vi "toml_example_load.vi"(8 "error in (no error)":errorcluster) -> (0 "error out":errorcluster)   [LabVIEW 2017]
panel:
  out "tables":variant
  in  "toml":string="################################################################################\n## Comment\n\n# Speak your mind with the hash symbol. They go from the symbol to the end of\n# the line.\n\n\n################################################################################\n## Table\n\n# Tables (also known as hash tables or dictionaries) are collections of\n# key/value pairs. They appear in square brackets on a line by themselves.\n\n[table]\n\nkey = \"value\" # Yeah, you can do this.\n\n# Nested tables are denoted by table names with dots in them. Name your tables\n# whatever crap you please, just don't use #, ., [ or ].\n\n[table.subtable]\n\nkey = \"another value\"\n\n# You don't need to specify all the super-tables if you don't want to. TOML\n# knows how to do it for you.\n\n# [x] you\n# [x.y] don't\n# [x.y.z] need these\n[x.y.z.w] # for this to work\n\n\n################################################################################\n## Inline Table\n\n# Inline tables provide a more compact syntax for expressing tables. They are\n# especially useful for grouped data that can otherwise quickly become verbose.\n# Inline tables are enclosed in curly braces `{` and `}`. No newlines are\n# allowed between the curly braces unless they are valid within a value.\n\n[table.inline]\n\nname = { first = \"Tom\", last = \"Preston-Werner\" }\npoint = { x = 1, y = 2 }\n\n\n################################################################################\n## String\n\n# There are four ways to express strings: basic, multi-line basic, literal, and\n# multi-line literal. All strings must contain only valid UTF-8 characters.\n\n[string.basic]\n\nbasic = \"I'm a string. \\\"You can quote me\\\". Name\\tJos\\u00E9\\nLocation\\tSF.\"\n\n[string.multiline]\n\n# The following strings are byte-for-byte equivalent:\nkey1 = \"One\\nTwo\"\nkey2 = \"\"\"One\\nTwo\"\"\"\nkey3 = \"\"\"\nOne\nTwo\"\"\"\n\n[string.multiline.continued]\n\n# The following strings are byte-for-byte equivalent:\nkey1 = \"The quick brown fox jumps over the lazy dog.\"\n\nkey2 = \"\"\"\nThe quick brown \\\n\n\n  fox jumps over \\\n    the lazy dog.\"\"\"\n\nkey3 = \"\"\"\\\n       The quick brown \\\n       fox jumps over \\\n       the lazy dog.\\\n       \"\"\"\n\n[string.literal]\n\n# What you see is what you get.\nwinpath  = 'C:\\Users\\nodejs\\templates'\nwinpath2 = '\\\\ServerX\\admin$\\system32\\'\nquoted   = 'Tom \"Dubs\" Preston-Werner'\nregex    = '<\\i\\c*\\s*>'\n\n\n[string.literal.multiline]\n\nregex2 = '''I [dw]on't need \\d{2} apples'''\nlines  = '''\nThe first newline is\ntrimmed in raw strings.\n   All other whitespace\n   is preserved.\n'''\n\n\n################################################################################\n## Integer\n\n# Integers are whole numbers. Positive numbers may be prefixed with a plus sign.\n# Negative numbers are prefixed with a minus sign.\n\n[integer]\n\nkey1 = +99\nkey2 = 42\nkey3 = 0\nkey4 = -17\n\n[integer.underscores]\n\n# For large numbers, you may use underscores to enhance readability. Each\n# underscore must be surrounded by at least one digit.\nkey1 = 1_000\nkey2 = 5_349_221\nkey3 = 1_2_3_4_5     # valid but inadvisable\n\n\n################################################################################\n## Float\n\n# A float consists of an integer part (which may be prefixed with a plus or\n# minus sign) followed by a fractional part and/or an exponent part.\n\n[float.fractional]\n\nkey1 = +1.0\nkey2 = 3.1415\nkey3 = -0.01\n\n[float.exponent]\n\nkey1 = 5e+22\nkey2 = 1e6\nkey3 = -2E-2\n\n[float.both]\n\nkey = 6.626e-34\n\n[float.underscores]\n\nkey1 = 9_224_617.445_991_228_313\nkey2 = 1e1_000\n\n\n################################################################################\n## Boolean\n\n# Booleans are just the tokens you're used to. Always lowercase.\n\n[boolean]\n\nTrue = true\nFalse = false\n\n\n################################################################################\n## Datetime\n\n# Datetimes are RFC 3339 dates.\n\n[datetime]\n\nkey1 = 1979-05-27T07:32:00Z\nkey2 = 1979-05-27T00:32:00-07:00\nkey3 = 1979-05-27T00:32:00.999999-07:00\n\n\n################################################################################\n## Array\n\n# Arrays are square brackets with other primitives inside. Whitespace is\n# ignored. Elements are separated by commas. Data types may not be mixed.\n\n[array]\n\nkey1 = [ 1, 2, 3 ]\nkey2 = [ \"red\", \"yellow\", \"green\" ]\nkey3 = [ [ 1, 2 ], [3, 4, 5] ]\nkey4 = [ [ 1, 2 ], [\"a\", \"b\", \"c\"] ] # this is ok\n\n# Arrays can also be multiline. So in addition to ignoring whitespace, arrays\n# also ignore newlines between the brackets.  Terminating commas are ok before\n# the closing bracket.\n\nkey5 = [\n  1, 2, 3\n]\nkey6 = [\n  1,\n  2, # this is ok\n]\n\n\n################################################################################\n## Array of Tables\n\n# These can be expressed by using a table name in double brackets. Each table\n# with the same double bracketed name will be an element in the array. The\n# tables are inserted in the order encountered.\n\n[[products]]\n\nname = \"Hammer\"\nsku = 738594937\n\n[[products]]\n\n[[products]]\n\nname = \"Nail\"\nsku = 284758393\ncolor = \"gray\"\n\n\n# You can create nested arrays of tables as well.\n\n[[fruit]]\n  name = \"apple\"\n\n  [fruit.physical]\n    color = \"red\"\n    shape = \"round\"\n\n  [[fruit.variety]]\n    name = \"red delicious\"\n\n  [[fruit.variety]]\n    name = \"granny smith\"\n\n[[fruit]]\n  name = \"banana\"\n\n  [[fruit.variety]]\n    name = \"plantain\""
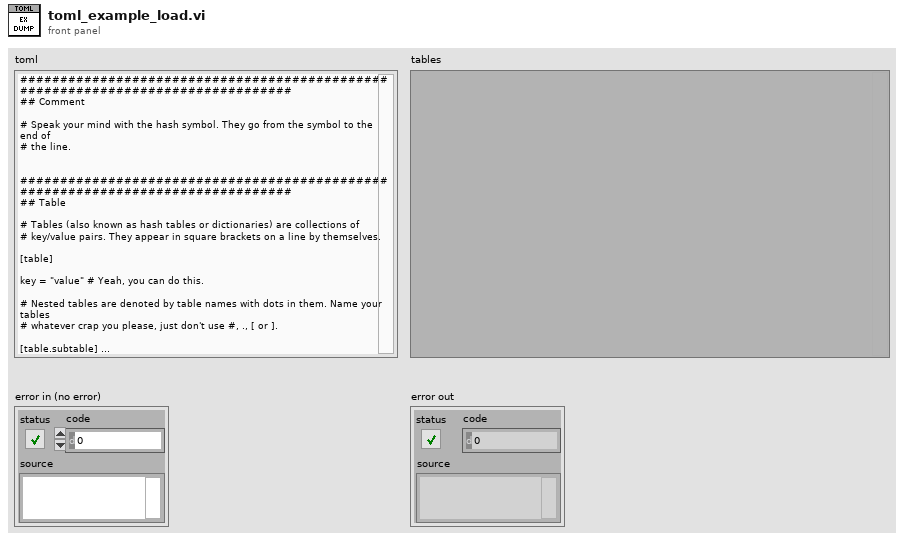
[diagram p1: front panel]
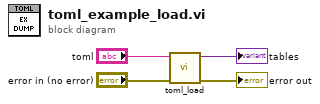
[diagram p0: block diagram]
diagram:
  n1 = call "toml_load.vi"("error in (no error)"="error in (no error)", "toml"="toml") -> ("error out"=→"error out":errorcluster, "tables"=→"tables":variant)  [unwired: 8 in]
